vi "Part 1.vi"(11 "Input":string) -> (3 "Output":i64)   [LabVIEW 2021]
uses:
  983c7286-f24c-4f8c-8ac8-876f989d8384.vi
panel:
  out "Array 2":cluster{"Valid Inputs":cluster{i32, i32}[]}[](array[cluster])
  in  "Runs":i32=6
  out "max value":i32
  out "Array":i32[](array[numeric])
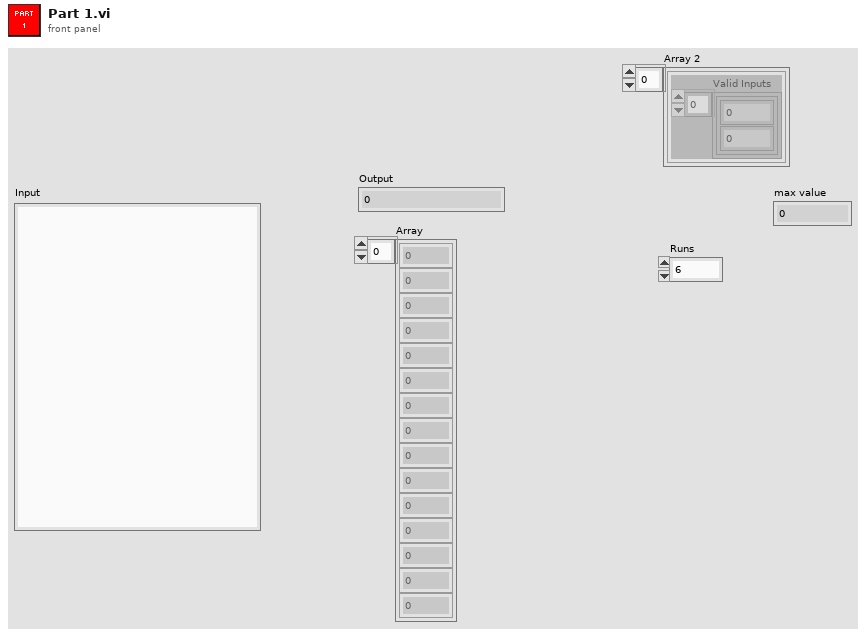
[diagram p1: front panel]
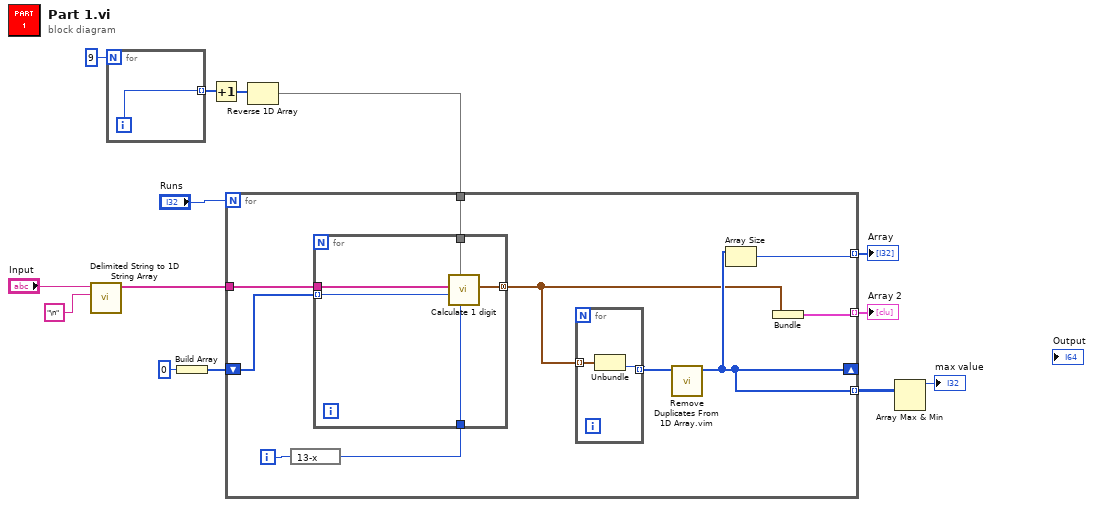
[diagram p0: block diagram]
diagram:
  n1 = call <vilib>:"Delimited String to 1D String Array.vi"("delimiter"="\n", "delimited string"="Input") -> ("string array"=w12:string[])  [unwired: 9 in]
  n2 = for {
    N: 9 -> [_]
    tunnel: [w15] -> w6 mode=indexing
    i -> [w15]
  }
  n3 = Build Array(i64 0 ("z in")) -> (w9:i64[])
  n4 = Increment(x=w6) -> (x+1=w5:i32[])
  n5 = Reverse 1D Array(array=w5) -> (reversed array=w4:i32[])
  n6 = for {
    N: "Runs" -> [_]
    tunnel: w12 -> [w25]
    shift-right: [w18] -> _
    shift-left: w9 -> [w24]
    tunnel: [w21] -> w8 mode=indexing
    tunnel: w4 -> [w20]
    tunnel: [w18] -> w3 mode=indexing
    tunnel: [w16] -> w1 mode=indexing
    i -> [w23]
    n7 = expression code="13-x"(w23) -> (w22:i32)
    n8 = for {
      tunnel: w25 -> [w32]
      tunnel: w24 -> [w31] mode=indexing
      tunnel: w22 -> [w30]
      tunnel: [w29] -> w17 mode=concatenating
      tunnel: w20 -> [w28]
      n9 = call "Calculate 1 digit.vi"("index"=w30, "Digits"=w28, "z out"=w31, "Input"=w32) -> ("Valid Inputs"=w29:cluster{i32, i32}[])  [unwired: 7 in]
    }
    n10 = for {
      tunnel: w17 -> [w27] mode=indexing
      tunnel: [w26] -> w19 mode=indexing
      n11 = Unbundle(w27) -> (w26:i32)  [unwired: 1 out]
    }
    n12 = call "Remove Duplicates From 1D Array.vim"("array"=w19) -> ("array with duplicates removed"=w18:i32[])  [unwired: 10 in]
    n13 = Array Size(array=w18) -> (size(s)=w21:i32)
    n14 = Bundle("Valid Inputs"=w17) -> (w16:cluster{"Valid Inputs":cluster{i32, i32}[]})  [unwired: 1 in]
  }
  "Array" <- w8
  "Array 2" <- w1
  n15 = Array Max & Min(array=w3) -> (max value=→"max value":i32)  [unwired: 3 out]
